vi "check_head_magic.vi"(3 "error in":errorcluster, 5 "refnum in":refnum<file>) -> (0 "error out":errorcluster, 2 "refnum out":refnum<file>)   [LabVIEW 2016]
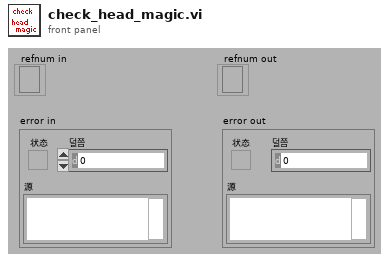
[diagram p1: front panel]
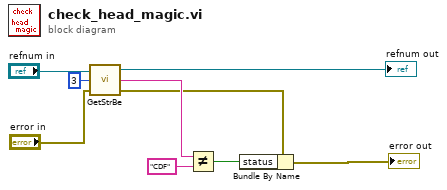
[diagram p0: block diagram]
diagram:
  n1 = call "GetStrBe.vi"("error in"="error in", "nchars"=3, "refnum in"="refnum in") -> ("error out"=w5:errorcluster, "str"=w7:string, "refnum out"=→"refnum out":refnum<file>)
  n2 = Not Equal?(x=w7, y="CDF") -> (x != y?=w4:bool)
  n3 = Bundle By Name(cluster=w5, "status"=w4) -> (→"error out":errorcluster)
